vi "Destroy_LV_INI_Token.vi"   [LabVIEW 2021]
uses:
  <vilib>/Wiresmith Technology/G CLI/CLI Class/CLI.lvclass
  <vilib>/Utility/config.llb/NI_LVConfig.lvlib
types:
  T1 = enum32{"Invalid", "Standard", "Closed", "Hidden", "Minimized", "Maximized"}
  T2 = typedef "NI_LVConfig.lvlib/Config Data RefNum.ctl" = refnum<k1>
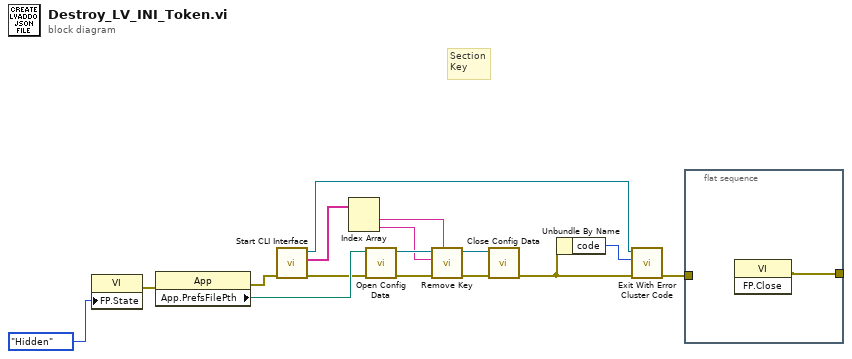
[diagram p0: block diagram]
diagram:
  # "Section\nKey"
  n1 = property class="VI"("FP.State"=T1."Hidden" ("Front Panel Window:State")) -> (error out=w12:errorcluster)  [unwired: 2 in, 1 out]
  n2 = property class="App"(error in=w12) -> (error out=w8:errorcluster, "App.PrefsFilePth"=w13:path)  [unwired: 1 in, 1 out]
  n3 = call <vilib>:"Start CLI Interface.vi"("error in (no error)"=w8) -> ("error out"=w9:errorcluster, "Custom Parameters"=w7:string[], "CLI out"=w14:refnum<class "CLI.lvclass">)  [unwired: 7 in, 1 out]
  n4 = Index Array(array=w7) -> (element #1=w2:string, element #2=w1:string)  [unwired: 2 in]
  n5 = call <vilib>:"Open Config Data.vi"("error in (no error)"=w9, "configuration file path"=w13) -> ("error out"=w6:errorcluster, "refnum"=w4:T2)  [unwired: 7 in, 1 out]
  n6 = call <vilib>:"Remove Key.vi"("section"=w2, "error in (no error)"=w6, "key"=w1, "refnum"=w4) -> ("error out"=w5:errorcluster, "refnum out"=w3:T2)  [unwired: 5 in, 1 out]
  n7 = call <vilib>:"Close Config Data.vi"("error in (no error)"=w5, "refnum"=w3) -> ("error out"=w11:errorcluster)  [unwired: 8 in, 1 out]
  n8 = Unbundle By Name(w11) -> ("code"=w10:i32)
  n9 = call <vilib>:"Exit With Error Cluster Code.vi"("error in (no error)"=w11, "No Error Code (0)"=w10, "CLI in"=w14) -> ("error out"=w15:errorcluster)  [unwired: 8 in]
  n10 = flat-sequence {
    tunnel: [w17] -> _
    tunnel: w15 -> [_]
    frame #0 {
      n11 = invoke class="VI" method="FP.Close"() -> (error out=w17:errorcluster)  [unwired: 3 in, 2 out]
    }
  }
